vi "GraphLockin_vs_Parameter.vi"(4 "V-":i32=1 min=1, 6 "V+":i32=1 min=1, 7 "reset?":bool, 8 "Current":i32=1 min=1, 9 "Parameter":dbl, 10 "Y[ ]":dbl[](array[numeric]), 11 "X[ ]":dbl[](array[numeric])) -> (0 "R(Ohms) vs Parameter":cluster{"Y":dbl[], "Y":dbl[]}[](graph), 1 "G(Siemens) vs Parameter":cluster{"Y":dbl[], "Y":dbl[]}[](graph), 2 "Y vs Parameter":cluster{dbl[], dbl[]}[](graph), 3 "X vs Parameter":cluster{dbl[], dbl[]}[](graph))   [LabVIEW 2019, in "Transport.lvclass"]
uses:
  Transport.lvclass
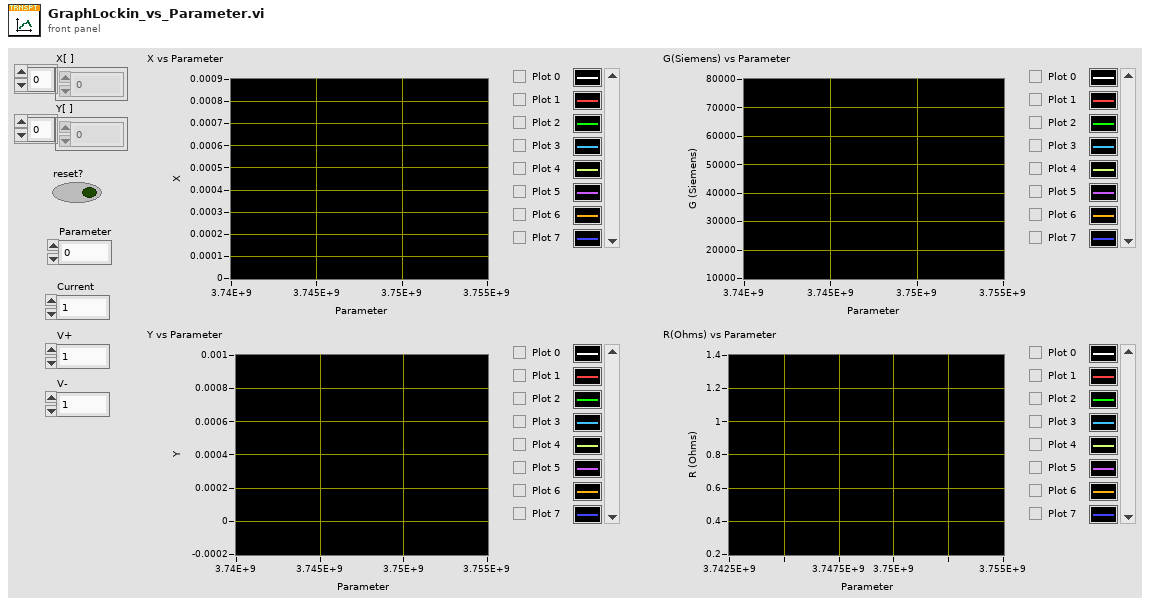
[diagram p1: front panel]
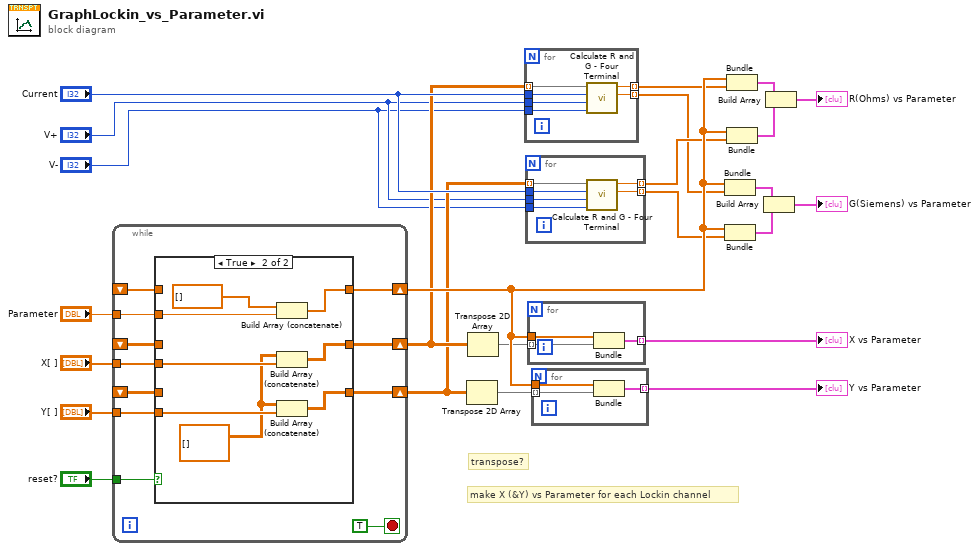
[diagram p0: block diagram]
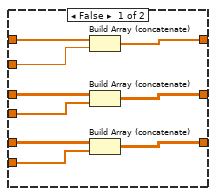
[diagram p2: hidden frame]
diagram:
  # "make X (&Y) vs Parameter for each Lockin channel"
  # "transpose?"
  n1 = while {
    tunnel: "X[ ]" -> [w35]
    tunnel: "Parameter" -> [w34]
    tunnel: "reset?" -> [w32]
    shift-right: [w25] -> w7
    shift-left: _ -> [w31]
    shift-right: [w26] -> w6
    shift-left: _ -> [w29]
    tunnel: "Y[ ]" -> [w30]
    shift-right: [w27] -> w13
    shift-left: _ -> [w28]
    stop <- TRUE stop-if-true
    n2 = case shown="True" w32 {
      tunnel: w35 -> [w37 w52]
      tunnel: w34 -> [w38 w47]
      tunnel: [w39 w49] -> w25
      tunnel: w31 -> [w44 _]
      tunnel: w30 -> [w36 w46]
      tunnel: w29 -> [w43 _]
      tunnel: [w40 w48] -> w26
      tunnel: [w41 w50] -> w27
      tunnel: w28 -> [w42 _]
      frame False {
        n3 = Build Array (concatenate)(w42, w38) -> (w41:dbl[])
        n4 = Build Array (concatenate)(w44, w37) -> (w39:dbl[][])
        n5 = Build Array (concatenate)(w43, w36) -> (w40:dbl[][])
      }
      frame True {
        w45 = dbl[][] []
        n6 = Build Array (concatenate)(dbl[] [], w47) -> (w50:dbl[])
        n7 = Build Array (concatenate)(w45, w52) -> (w49:dbl[][])
        n8 = Build Array (concatenate)(w45, w46) -> (w48:dbl[][])
      }
    }
  }
  n9 = Transpose 2D Array(2D array=w6) -> (transposed array=w8:dbl[][])
  n10 = Transpose 2D Array(2D array=w7) -> (transposed array=w9:dbl[][])
  n11 = for {
    tunnel: "Current" -> [w58]
    tunnel: "V+" -> [w57]
    tunnel: "V-" -> [w56]
    tunnel: [w55] -> w10 mode=indexing
    tunnel: w7 -> [w54] mode=indexing
    tunnel: [w53] -> w1 mode=indexing
    n12 = call "Calculate R and G - Four Terminal.vi"("V-"=w56, "V+"=w57, "Current"=w58, "Lockin[ ]"=w54) -> ("G_4T (Siemens)"=w53:dbl, "R_4T (ohms)"=w55:dbl)  [unwired: 4 in, 2 out]
  }
  n13 = for {
    tunnel: "Current" -> [w64]
    tunnel: "V+" -> [w63]
    tunnel: "V-" -> [w62]
    tunnel: [w60] -> w5 mode=indexing
    tunnel: w6 -> [w61] mode=indexing
    tunnel: [w59] -> w2 mode=indexing
    n14 = call "Calculate R and G - Four Terminal.vi"("V-"=w62, "V+"=w63, "Current"=w64, "Lockin[ ]"=w61) -> ("G_4T (Siemens)"=w59:dbl, "R_4T (ohms)"=w60:dbl)  [unwired: 4 in, 2 out]
  }
  n15 = for {
    tunnel: [w67] -> w20 mode=indexing
    tunnel: w13 -> [w66]
    tunnel: w9 -> [w65] mode=indexing
    n16 = Bundle(w66, w65) -> (w67:cluster{dbl[], dbl[]})  [unwired: 1 in]
  }
  "X vs Parameter" <- w20
  n17 = for {
    tunnel: [w70] -> w19 mode=indexing
    tunnel: w13 -> [w69]
    tunnel: w8 -> [w68] mode=indexing
    n18 = Bundle(w69, w68) -> (w70:cluster{dbl[], dbl[]})  [unwired: 1 in]
  }
  "Y vs Parameter" <- w19
  n19 = Bundle(w13, w1) -> (w18:cluster{dbl[], dbl[]})  [unwired: 1 in]
  n20 = Bundle(w13, w2) -> (w16:cluster{dbl[], dbl[]})  [unwired: 1 in]
  n21 = Bundle(w13, w10) -> (w14:cluster{dbl[], dbl[]})  [unwired: 1 in]
  n22 = Bundle(w13, w5) -> (w15:cluster{dbl[], dbl[]})  [unwired: 1 in]
  n23 = Build Array(w18, w16) -> (→"G(Siemens) vs Parameter":cluster{dbl[], dbl[]}[])
  n24 = Build Array(w14, w15) -> (→"R(Ohms) vs Parameter":cluster{dbl[], dbl[]}[])
